vi "GEA3 Inverter ERDs.vi"(8 "error in":errorcluster, 10 "Inverter  ERD Data":T3[](array[typedef]) {"ERD Number" format="%.0x"}, 11 "ERD Data":T1) -> (0 "error out":errorcluster, 3 "ERD Data Output":T1, 5 "Inverter Data":string[][](array[string]))   [LabVIEW 2023]
uses:
  type defs/ERD Read Data Out.ctl
  Type Definitions/GEA3 HEWH ERD Data.ctl
  Type Definitions/GEA3 HEWH Mixing Valve.ctl
  library/GEA2_Toolkit.lvlib
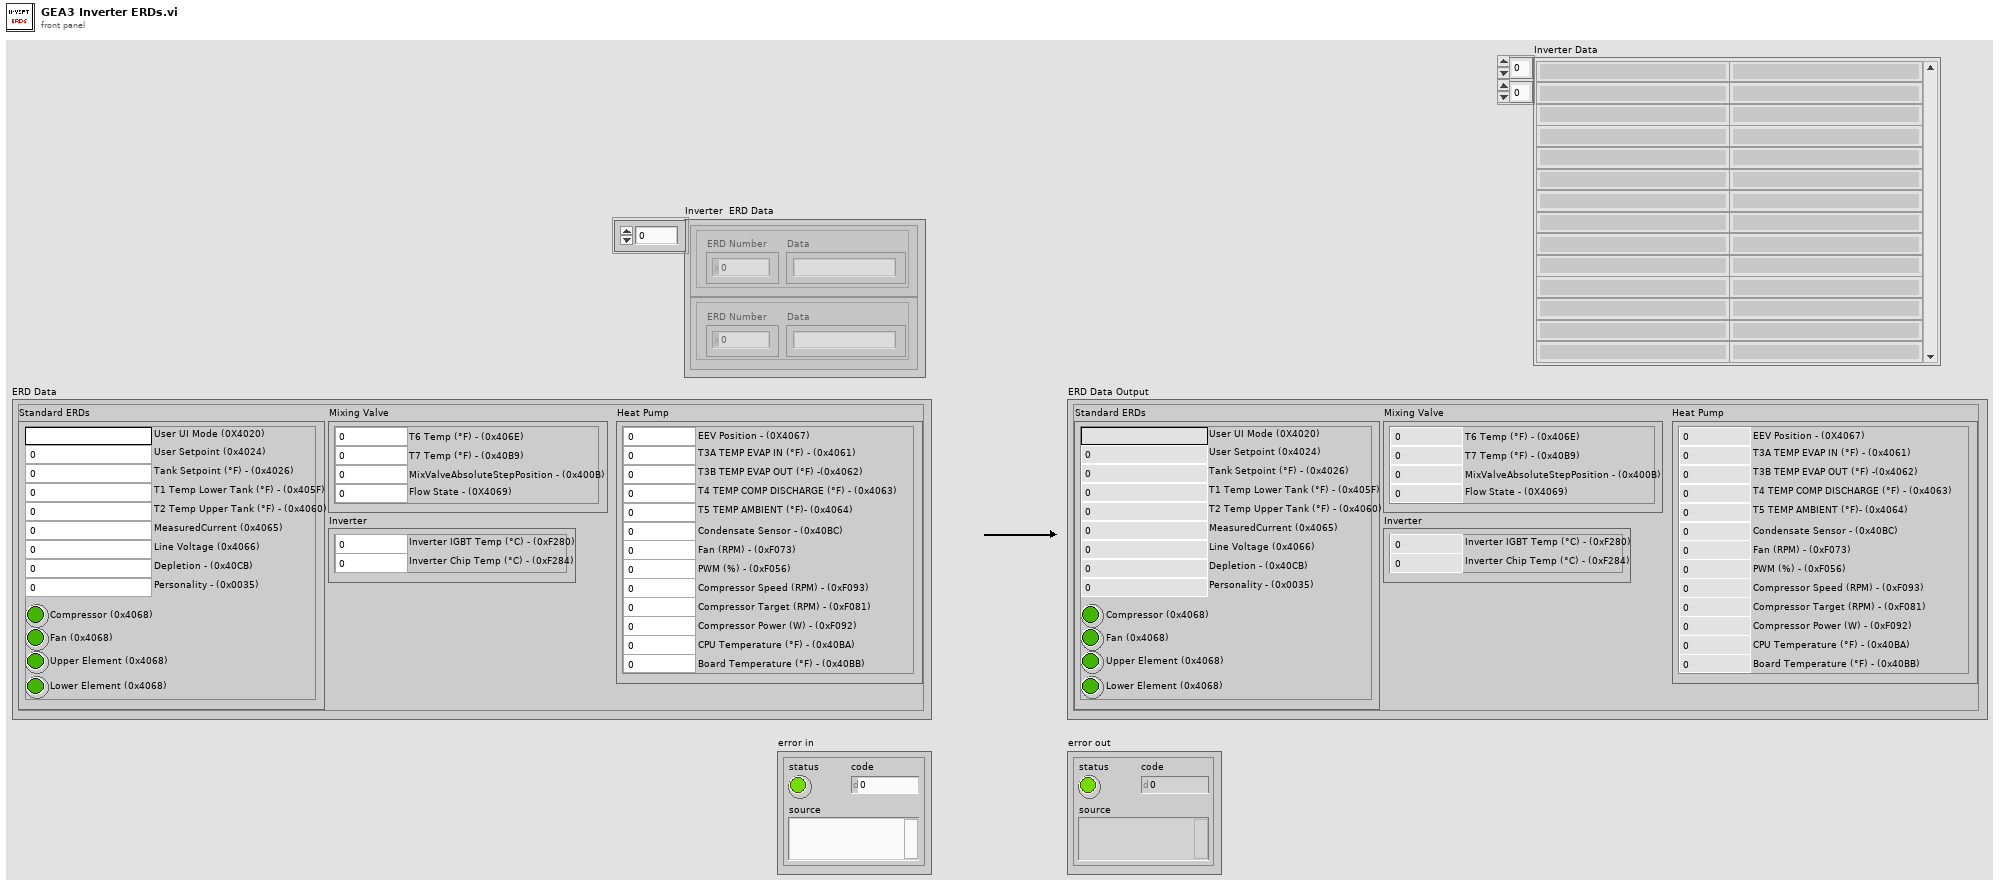
[diagram p1: front panel]
types:
  T1 = typedef "GEA3 HEWH ERD Data.ctl" = cluster{"Mixing Valve":T2, "Standard ERDs":cluster{"User UI Mode (0X4020)":string, "User Setpoint (0x4024)":u16, "Compressor (0x4068)":bool, "Lower Element (0x4068)":bool, "Upper Element (0x4068)":bool, "Fan (0x4068)":bool, "T1 Temp Lower Tank (°F) - (0x405F)":dbl, "T2 Temp Upper Tank (°F) - (0x4060)":dbl, "Line Voltage (0x4066)":u16, "MeasuredCurrent (0x4065)":dbl, "Tank Setpoint (°F) - (0x4026)":u16, "Depletion - (0x40CB)":u16, "Personality - (0x0035)":u16}, "Heat Pump":cluster{"EEV Position - (0X4067)":u16, "T3A TEMP EVAP IN (°F) - (0x4061)":dbl, "T3B TEMP EVAP OUT (°F) -(0x4062)":dbl, "T4 TEMP COMP DISCHARGE (°F) - (0x4063)":dbl, "T5 TEMP AMBIENT (°F)- (0x4064)":dbl, "Condensate Sensor - (0x40BC)":u16, "Fan (RPM) - (0xF073)":u16, "PWM (%) - (0xF056)":u16, "Compressor Speed (RPM) - (0xF093)":u16, "Compressor Target (RPM) - (0xF081)":u16, "Compressor Power (W) - (0xF092)":u16, "CPU Temperature (°F) - (0x40BA)":dbl, "Board Temperature (°F) - (0x40BB)":dbl}, "Inverter":cluster{"Inverter IGBT Temp (°C) - (0xF280)":dbl, "Inverter Chip Temp (°C) - (0xF284)":dbl}}
  T2 = typedef "GEA3 HEWH Mixing Valve.ctl" = cluster{"T7 Temp (°F) - (0x40B9)":dbl, "MixValveAbsoluteStepPosition - (0x400B)":i16, "Flow State - (0X4069)":u8, "T6 Temp (°F) - (0x406E)":dbl}
  T3 = typedef "GEA2_Toolkit.lvlib/ERD Read Data Out.ctl" = cluster{"ERD Number":u16, "Data":string}
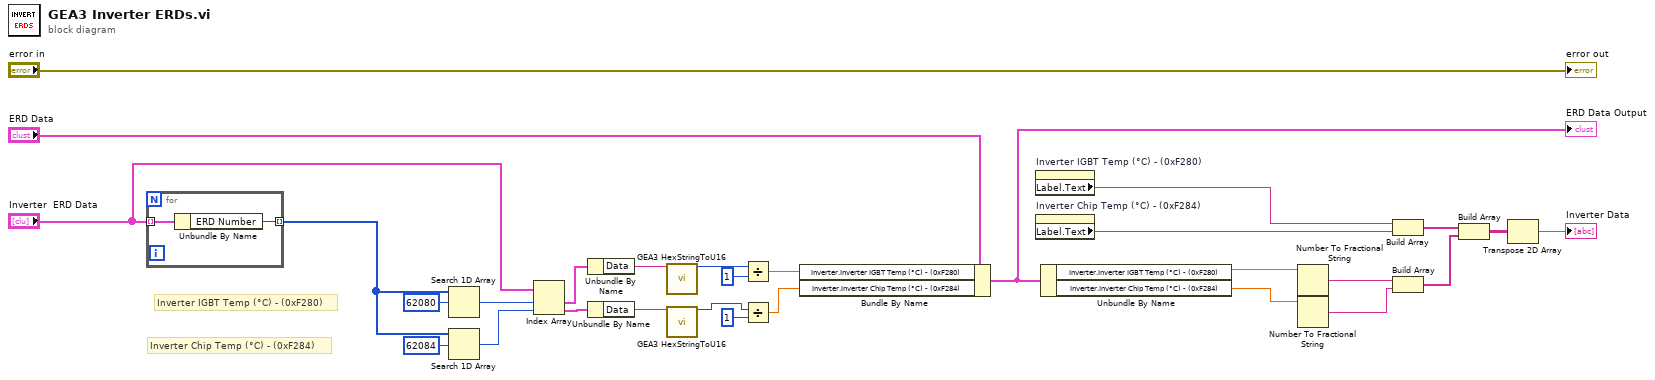
[diagram p0: block diagram]
diagram:
  # "Inverter Chip Temp (°C) - (0xF284)"
  # "Inverter IGBT Temp (°C) - (0xF280)"
  n1 = for {
    tunnel: "Inverter  ERD Data" -> [w31] mode=indexing
    tunnel: [w30] -> w29 mode=indexing
    n2 = Unbundle By Name(w31) -> ("ERD Number"=w30:u16)
  }
  n3 = Search 1D Array(1D array=w29, element=u16 62080 ("ERD Number")) -> (index of element=w13:i32)  [unwired: 1 in]
  n4 = Search 1D Array(1D array=w29, element=u16 62084 ("ERD Number")) -> (index of element=w14:i32)  [unwired: 1 in]
  n5 = Index Array(array="Inverter  ERD Data", index #1=w13, index #2=w14) -> (element #1=w18:T3, element #2=w17:T3)
  n6 = Unbundle By Name(w18) -> ("Data"=w15:string)
  n7 = Unbundle By Name(w17) -> ("Data"=w16:string)
  n8 = call "GEA3 HexStringToU16.vi"("Input String"=w15) -> ("Number Out"=w20:u16)  [unwired: 14 in]
  n9 = call "GEA3 HexStringToU16.vi"("Input String"=w16) -> ("Number Out"=w22:u16)  [unwired: 14 in]
  n10 = Divide(x=w20, y=u16 1) -> (x/y=w23:dbl)
  n11 = Divide(x=w22, y=u16 1) -> (x/y=w24:dbl)
  n12 = Bundle By Name(cluster="ERD Data", "Inverter.Inverter IGBT Temp (°C) - (0xF280)"=w23, "Inverter.Inverter Chip Temp (°C) - (0xF284)"=w24) -> (w5:T1)
  "ERD Data Output" <- w5
  n13 = property on="Inverter IGBT Temp (°C) - (0xF280)" class="DigNum (strict)"() -> ("Label.Text"=w2:string)  [unwired: 2 in, 2 out]
  n14 = property on="Inverter Chip Temp (°C) - (0xF284)" class="DigNum (strict)"() -> ("Label.Text"=w1:string)  [unwired: 2 in, 2 out]
  n15 = Unbundle By Name(w5) -> ("Inverter.Inverter IGBT Temp (°C) - (0xF280)"=w25:dbl, "Inverter.Inverter Chip Temp (°C) - (0xF284)"=w26:dbl)
  n16 = Number To Fractional String(number=w25) -> (F-format string=w27:string)  [unwired: 3 in]
  n17 = Number To Fractional String(number=w26) -> (F-format string=w28:string)  [unwired: 3 in]
  n18 = Build Array(w2, w1) -> (w10:string[])
  n19 = Build Array(w27, w28) -> (w9:string[])
  n20 = Build Array(w10, w9) -> (w8:string[][])
  n21 = Transpose 2D Array(2D array=w8) -> (transposed array=→"Inverter Data":string[][])
  "error out" <- "error in"
